vi "Shooter.vi"(0 "Shoot":bool, 1 "Reverse shooter + Feeder":bool, 2 "Feed Shooter":bool, 3 "Reverse Swirly":bool) -> ()   [LabVIEW 2016]
uses:
  <vilib>/Rock Robotics/WPI/ThirdParty/CanMotor/TalonSRX/WPI_CANTalonSRX_APIFeedbackSelect.ctl
  <vilib>/Rock Robotics/WPI/ThirdParty/CanMotor/TalonSRX/WPI_CANTalonSRX_APIControlMode.ctl
panel:
  in  "Feeder %":dbl(slide)=0.9 scale=0.0..1.0
  in  "Shooter PIDF":T1={"P"=0.0, "I"=0.0001, "D"=0.0, "F"=0.0, "I Zone"=0.0, "Ramp Rate"=1.2}
  in  "Target RPM":dbl(slide)=0.556786703601108 scale=0.0..1.0
  in  "Swirly %":dbl(slide)=0.8 scale=0.0..1.0
  in  "Reverse Closed-Loop Output":bool
  in  "Reverse Feedback Sensor":bool
  out "Motor output Plot":cluster{"Applied Throttle":dbl}(graph)
  out "Speed Closed Loop Plots":cluster{dbl, "Sensor Velocity":dbl}(graph)
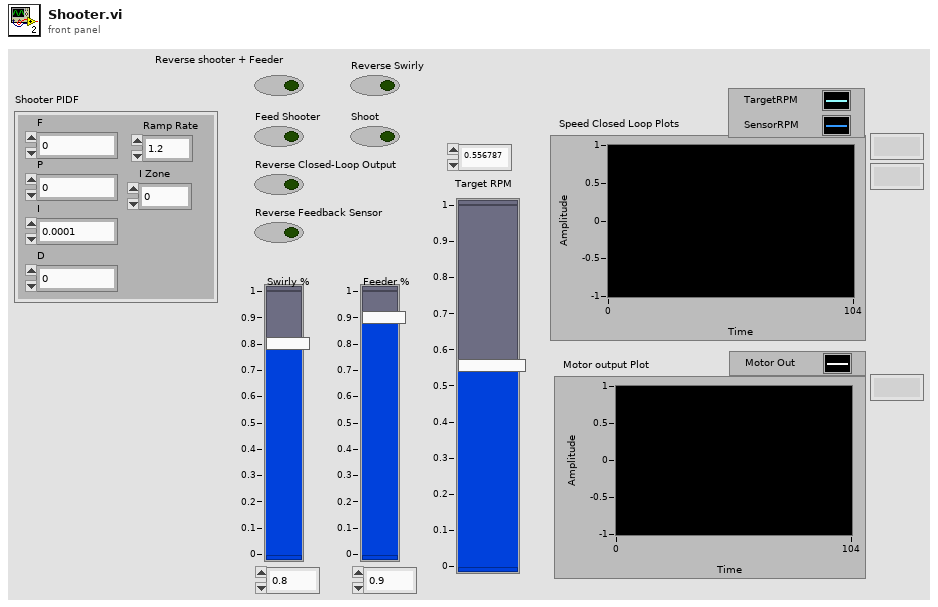
[diagram p1: front panel]
types:
  T1 = cluster{"P":dbl, "I":dbl, "D":dbl, "F":dbl, "I Zone":dbl, "Ramp Rate":dbl}
  T2 = typedef "WPI_CANTalonSRX_APIFeedbackSelect.ctl" = enum16{"Digital Quadrature Encoder", "Analog Potentiometer", "Analog Encoder", "Count on Quad-A (Rising-Edge)", "Count on Quad-A (Falling-Edge)", "CTR Magnetic Enc (Absolute)", "CTR Magnetic Enc (Relative)", "Pulse Width"}
  T3 = typedef "WPI_CANTalonSRX_APIControlMode.ctl" = enum8{"Percent VBus", "Speed", "Position", "Slave", "Unchanged / Invalid", "Voltage Compensation", "Current", "Motion Profile", "Motion Magic"}
  T4 = typedef "WPI_MotorControlDeviceRef.ctl" = cluster{"DeviceStatus":errorcluster, "Type":T5, "PWM":cluster{"PWM Channel":T6, "DeadBand":T7}, "CAN":cluster{"Device Number":u8, "SetOutput VI Ref":variant, "GetOutput VI Ref":variant, "Enable VI Ref":variant, "Disable VI Ref":variant, "Data":variant}, "Invert":bool}
  T5 = typedef "WPI_MotorControlType.ctl" = enum16{"PWM", "CAN"}
  T6 = typedef "FPGA_DIOPWMChannel.ctl" = enum8{"PWM 0", "PWM 1", "PWM 2", "PWM 3", "PWM 4", "PWM 5", "PWM 6", "PWM 7", "PWM 8", "PWM 9", "PWM MXP 0", "PWM MXP 1", "PWM MXP 2", "PWM MXP 3", "PWM MXP 4", "PWM MXP 5", "PWM MXP 6", "PWM MXP 7", "PWM MXP 8", "PWM MXP 9", "Invalid"}
  T7 = typedef "WPI_PWMDeadband.ctl" = cluster{"Name":string, "maxPositivePwm":i32, "minPositivePwm":i32, "centerPwm":i32, "maxNegativePwm":i32, "minNegativePwm":i32, "angularRange":u16}
  T8 = typedef "WPI_CANTalonSRX_GlobalStatus.ctl" = cluster{"Applied Throttle":dbl, "Module Enabled":bool, "CAN Error":errorcluster, "Closed Loop Error":dbl, "Forward Limit Switch Closed":bool, "Reverse Limit Switch Closed":bool, "Sensor Position":dbl, "Sensor Velocity":dbl, "Current":dbl, "Sticky Fault - Over Temp":bool, "Sticky Fault - Under Voltage":bool, "Sticky Fault - Forward Limit":bool, "Sticky Fault - Reverse Limit":bool, "Sticky Fault - Forward Soft Limit":bool, "Sticky Fault - Reverse Soft Limit":bool, "Brake is Enabled":bool, "Encoder Position":dbl, "Encoder Velocity":dbl, "Encoder Index Count":dbl, "Encoder A Pin State":bool, "Encoder B Pin State":bool, "Encoder Index Pin State":bool, "Analog In":dbl, "Analog In Velocity":dbl, "Temperature (C)":dbl, "Battery Voltage":dbl, "Control 5 Is Supported":bool, "Current Profile Slot Select":dbl, "Pos Div 8":bool, "Vel Div 4":bool, "Pulse Width Position":i32, "Pulse Width Velocity":i32, "Pulse Width Rise To Rise (us)":i32, "Pulse Width Rise To Fall (us)":i32, "Mot Prof Active Is Under Run":bool, "Mot Prof Active Has Under Run":bool, "Mot Prof Active Is Last":bool, "Mot Prof Active Velocity Only":bool, "Mot Prof Active Is Valid":bool, "Mot Prof Buffer Is Full":bool, "Mot Prof Active Profile Slot Select":i32, "Mot Prof NextID":i32, "Mot Prof Count":i32, "Mot Prof Active Velocity":dbl, "Mot Prof Active Position":dbl, "Mot Prof Output Enable":i32, "UsageFrame":u32}
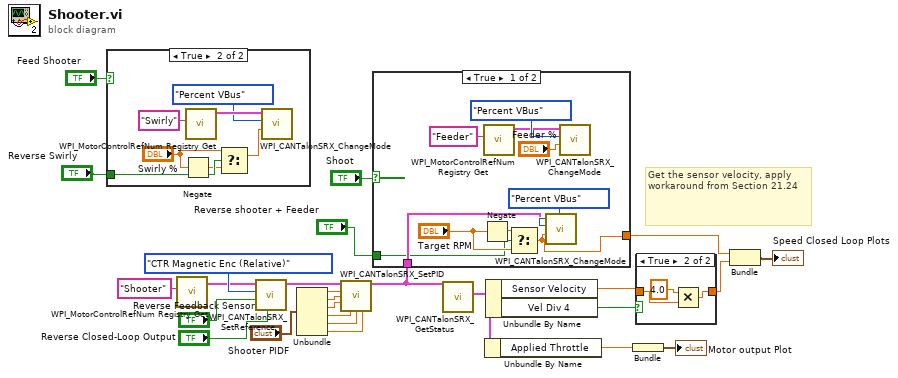
[diagram p0: block diagram]
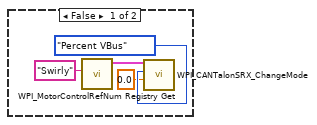
[diagram p2: hidden frame]
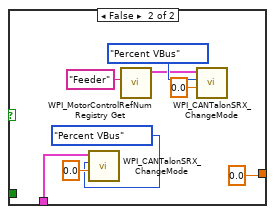
[diagram p3: hidden frame]
diagram:
  # "Get the sensor velocity, apply workaround from Section 21.24"
  n1 = case shown="True" "Feed Shooter" {
    tunnel: "Reverse Swirly" -> [_ w33]
    frame False {
      n2 = call <vilib>:"WPI_MotorControlRefNum Registry Get.vi"("refnum name"="Swirly") -> ("MotorControlDevRef"=w29:T4)  [unwired: 9 in, 1 out]
      n3 = call <vilib>:"WPI_CANTalonSRX_ChangeMode.vi"("Output"=0.0, "Control Mode"=WPI_CANTalonSRX_APIControlMode."Percent VBus", "CAN Talon SRX Ref"=w29) -> ()  [unwired: 7 in, 2 out]
    }
    frame True {
      n4 = Negate(x="Swirly %") -> (-x=w31:dbl)
      n5 = call <vilib>:"WPI_MotorControlRefNum Registry Get.vi"("refnum name"="Swirly") -> ("MotorControlDevRef"=w37:T4)  [unwired: 9 in, 1 out]
      n6 = Select(t="Swirly %", s=w33, f=w31) -> (s? t:f=w34:dbl)
      n7 = call <vilib>:"WPI_CANTalonSRX_ChangeMode.vi"("Output"=w34, "Control Mode"=WPI_CANTalonSRX_APIControlMode."Percent VBus", "CAN Talon SRX Ref"=w37) -> ()  [unwired: 7 in, 2 out]
    }
  }
  n8 = call <vilib>:"WPI_MotorControlRefNum Registry Get.vi"("refnum name"="Shooter") -> ("MotorControlDevRef"=w22:T4)  [unwired: 9 in, 1 out]
  n9 = call <vilib>:"WPI_CANTalonSRX_SetReference.vi"("Reverse Closed-Loop Output"="Reverse Closed-Loop Output", "Reverse Feedback Sensor"="Reverse Feedback Sensor", "Feedback Reference"=WPI_CANTalonSRX_APIFeedbackSelect."CTR Magnetic Enc (Relative)" ("Feedback Reference Shooter"), "CAN Talon SRX Ref"=w22) -> ("CAN Talon SRX Ref"=w21:T4)  [unwired: 6 in, 1 out]
  n10 = Unbundle("Shooter PIDF") -> ("P"=w10:dbl, "I"=w9:dbl, "D"=w8:dbl, "F"=w7:dbl, "I Zone"=w6:dbl, "Ramp Rate"=w5:dbl)
  n11 = call <vilib>:"WPI_CANTalonSRX_SetPID.vi"("CAN Talon SRX Ref"=w21, "P"=w10, "I"=w9, "D"=w8, "F"=w7, "I Zone"=w6, "Ramp Rate"=w5) -> ("CAN Talon SRX Ref"=w18:T4)  [unwired: 7 in, 1 out]
  n12 = case shown="True" "Shoot" {
    tunnel: w18 -> [w46 w53]
    tunnel: [w39 0.0 ("x")] -> w13
    tunnel: "Reverse shooter + Feeder" -> [w38 _]
    frame True {
      n13 = Negate(x="Target RPM") -> (-x=w40:dbl)
      n14 = call <vilib>:"WPI_MotorControlRefNum Registry Get.vi"("refnum name"="Feeder") -> ("MotorControlDevRef"=w42:T4)  [unwired: 9 in, 1 out]
      n15 = Select(t=w40, s=w38, f="Target RPM") -> (s? t:f=w39:dbl)
      n16 = call <vilib>:"WPI_CANTalonSRX_ChangeMode.vi"("Output"=w39, "Control Mode"=WPI_CANTalonSRX_APIControlMode."Percent VBus", "CAN Talon SRX Ref"=w46) -> ()  [unwired: 7 in, 2 out]
      n17 = call <vilib>:"WPI_CANTalonSRX_ChangeMode.vi"("Output"="Feeder %", "Control Mode"=WPI_CANTalonSRX_APIControlMode."Percent VBus", "CAN Talon SRX Ref"=w42) -> ()  [unwired: 7 in, 2 out]
    }
    frame False {
      n18 = call <vilib>:"WPI_CANTalonSRX_ChangeMode.vi"("Output"=0.0, "Control Mode"=WPI_CANTalonSRX_APIControlMode."Percent VBus", "CAN Talon SRX Ref"=w53) -> ()  [unwired: 7 in, 2 out]
      n19 = call <vilib>:"WPI_MotorControlRefNum Registry Get.vi"("refnum name"="Feeder") -> ("MotorControlDevRef"=w50:T4)  [unwired: 9 in, 1 out]
      n20 = call <vilib>:"WPI_CANTalonSRX_ChangeMode.vi"("Output"=0.0, "Control Mode"=WPI_CANTalonSRX_APIControlMode."Percent VBus", "CAN Talon SRX Ref"=w50) -> ()  [unwired: 7 in, 2 out]
    }
  }
  n21 = call <vilib>:"WPI_CANTalonSRX_GetStatus.vi"("CAN Talon SRX Ref"=w18) -> ("Talon SRX Status"=w19:T8)  [unwired: 8 in, 2 out]
  n22 = Unbundle By Name(w19) -> ("Applied Throttle"=w16:dbl)
  n23 = Unbundle By Name(w19) -> ("Sensor Velocity"=w24:dbl, "Vel Div 4"=w23:bool)
  n24 = Bundle("Applied Throttle"=w16) -> (→"Motor output Plot":cluster{"Applied Throttle":dbl})  [unwired: 1 in]
  n25 = case shown="True" w23 {
    tunnel: [w56 w58] -> w12
    tunnel: w24 -> [w56 w57]
    frame False {
    }
    frame True {
      n26 = Multiply(x=4.0, y=w57) -> (x*y=w58:dbl)
    }
  }
  n27 = Bundle("x"=w13, "Sensor Velocity"=w12) -> (→"Speed Closed Loop Plots":cluster{"x":dbl, "Sensor Velocity":dbl})  [unwired: 1 in]
